vi "NI VeriStand - Create and Load Runtime Configuration File.vi"(6 "File Path":string, 7 "Version":string, 8 "Error in":errorcluster, 9 "Creator":string, 10 "Description":string, 11 "Name":string) -> (0 "Error out":errorcluster, 2 "Base Section ID":u64, 3 "Runtime Configuration Ref":refnum<k39>)   [LabVIEW 2027, in "Runtime Configuration File API.lvlib"]
uses:
  Runtime Configuration File API.lvlib
  C:/NetCoreDLL/NationalInstruments.VeriStand.SystemDefinitionAPI.dll
  NetCoreDLL/NationalInstruments.VeriStand.SystemDefinitionAPI.dll
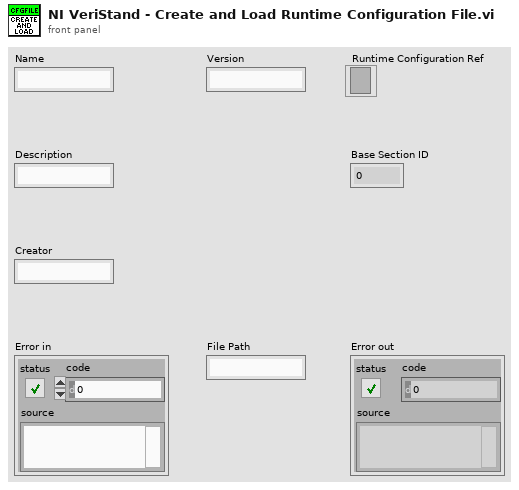
[diagram p1: front panel]
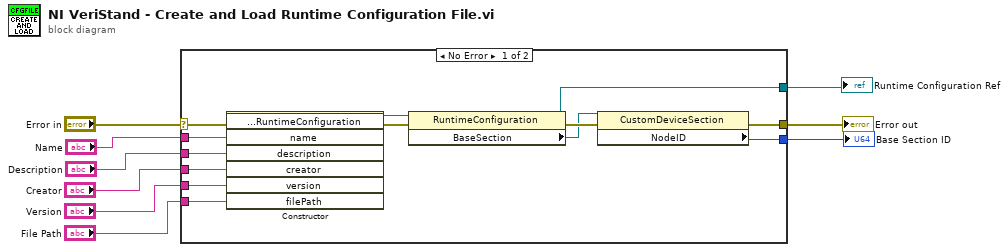
[diagram p0: block diagram]
diagram:
  n1 = case shown="No Error" "Error in" {
    selector: "Error in" -> [w22 w23]
    tunnel: "Name" -> [w18 _]
    tunnel: "Description" -> [w17 _]
    tunnel: "Creator" -> [w16 _]
    tunnel: "Version" -> [w15 _]
    tunnel: "File Path" -> [w14 _]
    tunnel: [w19 w23] -> w9
    tunnel: [w12 _] -> w2
    tunnel: [w11 _] -> w1
    frame No Error {
      n2 = constructor class="RuntimeConfiguration"(error in=w22, "name"=w18, "description"=w17, "creator"=w16, "version"=w15, "filePath"=w14) -> (reference out=w13:refnum<k39>, error out=w21:errorcluster)  [unwired: 2 in, 6 out]
      n3 = property class="RuntimeConfiguration"(reference=w13, error in=w21) -> (reference out=w12:refnum<k39>, error out=w20:errorcluster, "BaseSection"=w10:refnum<k39>)
      n4 = property class="CustomDeviceSection"(reference=w10, error in=w20) -> (error out=w19:errorcluster, "NodeID"=w11:u64)  [unwired: 1 out]
    }
    frame Error {
    }
  }
  "Runtime Configuration Ref" <- w2
  "Error out" <- w9
  "Base Section ID" <- w1
